vi "onCreate.vi"(8 "error in (no error)":errorcluster, 11 "SMO.Dictionary.Variant":refnum<class "SMO.Dictionary.Variant.lvclass">) -> (0 "error out":errorcluster, 3 "SMO.Dictionary.Variant out":refnum<class "SMO.Dictionary.Variant.lvclass">)   [LabVIEW 2013, in "SMO.Dictionary.lvlib" / "SMO.Dictionary.Variant.lvclass"]
doc: "JKI State Machine Objects (SMO) 1.0.1.12\nJKI - JKI\nCopyright (c) 2016, JKI"
uses:
  SMO.Dictionary.Variant.lvclass
  SMO.Dictionary.Variant.lvclass/SMO.Dictionary.Variant.ctl
  SMO.Dictionary/SMO.Dictionary.lvclass
panel:
  # "For instructions on how to use the JKI State Machine Objects, examples and video tutorials, visit:\nhttp://jki.net/state-machine-objects/\n\nJKI State Machine Objects™\nhttp://jki.net/state-machine-objects/\nCopyright (C) 2005-2015, JKI <info@jki.net>\nALL RIGHTS RESERVED"
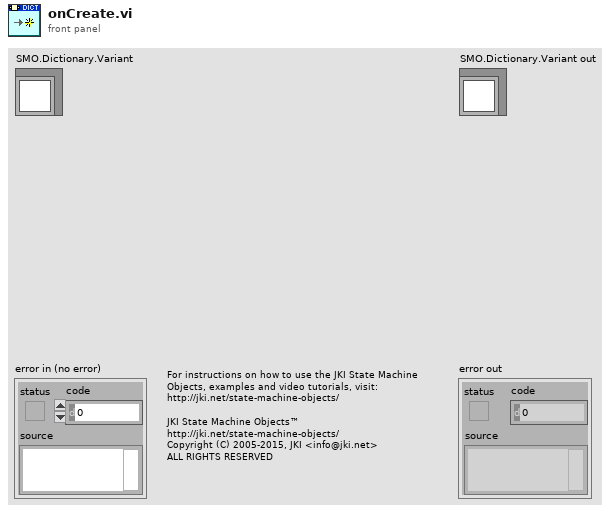
[diagram p1: front panel]
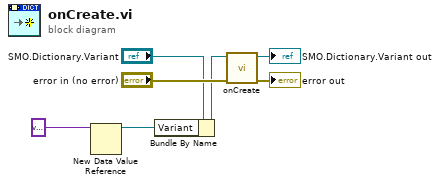
[diagram p0: block diagram]
diagram:
  n1 = New Data Value Reference(data value=variant ("Variant")) -> (data value reference=w1:refnum<data-value>)  [unwired: 1 in, 1 out]
  n2 = Bundle By Name(cluster="SMO.Dictionary.Variant", "Variant"=w1) -> (w3:refnum<class "SMO.Dictionary.Variant.lvclass">)
  n3 = call-parent "onCreate.vi"("error in (no error)"="error in (no error)", "SMO"=w3) -> ("error out"=→"error out":errorcluster, "SMO out"=→"SMO.Dictionary.Variant out":refnum<class "SMO.Dictionary.Variant.lvclass">)  [unwired: 8 in]
